vi "Bulid Status List.vi"(8 "Array in":string[](array[string]), 11 "Text.Text":string) -> (3 "Array":cluster{"Status":string, "InState":string}[](array[cluster]))   [LabVIEW 2017, in "CSM-Helper.lvclass"]
uses:
  CSM-Helper.lvclass
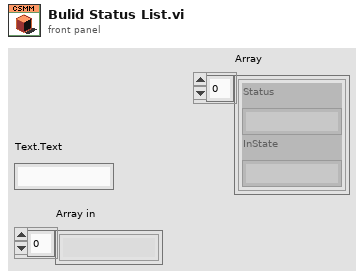
[diagram p1: front panel]
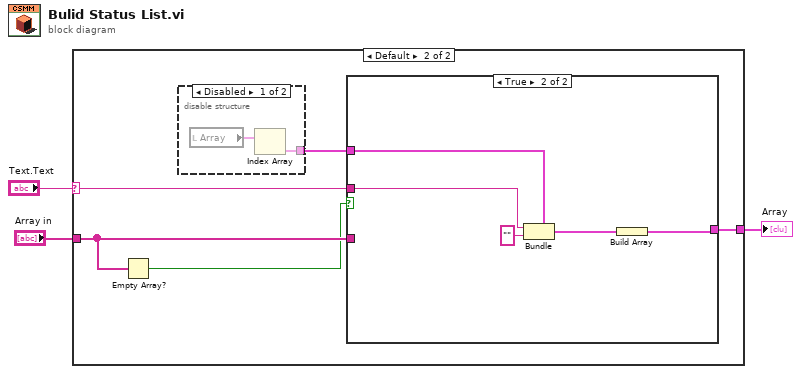
[diagram p0: block diagram]
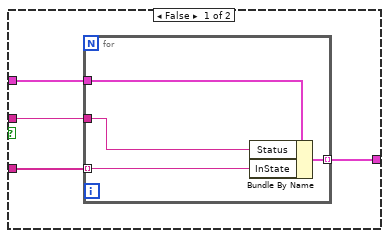
[diagram p4: hidden frame]
diagram:
  n1 = case shown="Default" "Text.Text" {
    selector: "Text.Text" -> [_ w8]
    tunnel: [_ w7] -> w2
    tunnel: "Array in" -> [_ w6]
    frame "" {
    }
    frame Default {
      n2 = Empty Array?(array=w6) -> (empty?=w5:bool)
      n3 = disable-structure shown="Disabled" {
        disable-tunnel: [w10 _] -> w4
        frame Disabled {
          n4 = local read "Array"() -> (w9:cluster{"Status":string, "InState":string}[])
          n5 = Index Array(array=w9) -> (element=w10:cluster{"Status":string, "InState":string})  [unwired: 1 in]
        }
        frame Enabled {
        }
      }
      n6 = case shown="True" w5 {
        tunnel: w8 -> [w14 w22]
        tunnel: [w13 w19] -> w7
        tunnel: w6 -> [w12 _]
        tunnel: w4 -> [w11 w23]
        frame False {
          n7 = for {
            tunnel: w14 -> [w18]
            tunnel: [w17] -> w13 mode=indexing
            tunnel: w12 -> [w16] mode=indexing
            tunnel: w11 -> [w15]
            n8 = Bundle By Name(cluster=w15, "Status"=w18, "InState"=w16) -> (w17:cluster{"Status":string, "InState":string})
          }
        }
        frame True {
          n9 = Bundle(cluster=w23, "Status"=w22, "InState"="") -> (w20:cluster{"Status":string, "InState":string})
          n10 = Build Array(w20) -> (w19:cluster{"Status":string, "InState":string}[])
        }
      }
    }
  }
  "Array" <- w2
